vi "Apply Disabled.vi"(8 "error in (no error)":errorcluster, 10 "Disabled":bool, 11 "BluelinesRedlines in":refnum<class "BluelinesRedlines.lvclass">) -> (0 "error out":errorcluster, 3 "BluelinesRedlines out":refnum<class "BluelinesRedlines.lvclass">)   [LabVIEW 2020, in "VolatusGUIElements.lvlib" / "BluelinesRedlines.lvclass"]
uses:
  BluelinesRedlines.lvclass
  BluelinesRedlines.lvclass/BluelinesRedlines.ctl
  VolatusGUI/GUI Element/GUI Element.lvclass
  C:/dev/lv20CE/relink/lv-volatus/VolatusGUI/GUI Element/GUI Element.lvclass
  C:/dev/lv20CE/relink/lv-volatus/VolatusGUIElements/BluelinesRedlines/BluelinesRedlines.lvclass
  C:/dev/lv20CE/relink/lv-volatus/VolatusGUI/OnValueChangeHandler/OnValueChangeHandler.lvclass
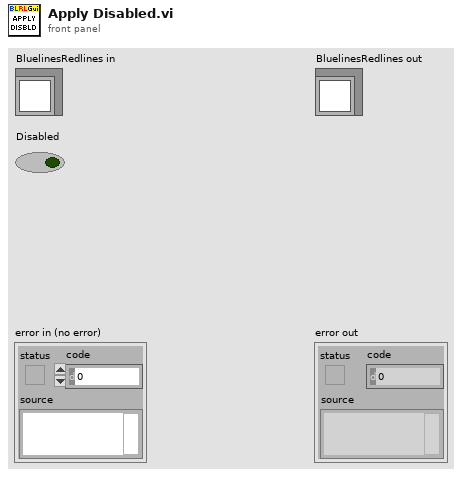
[diagram p1: front panel]
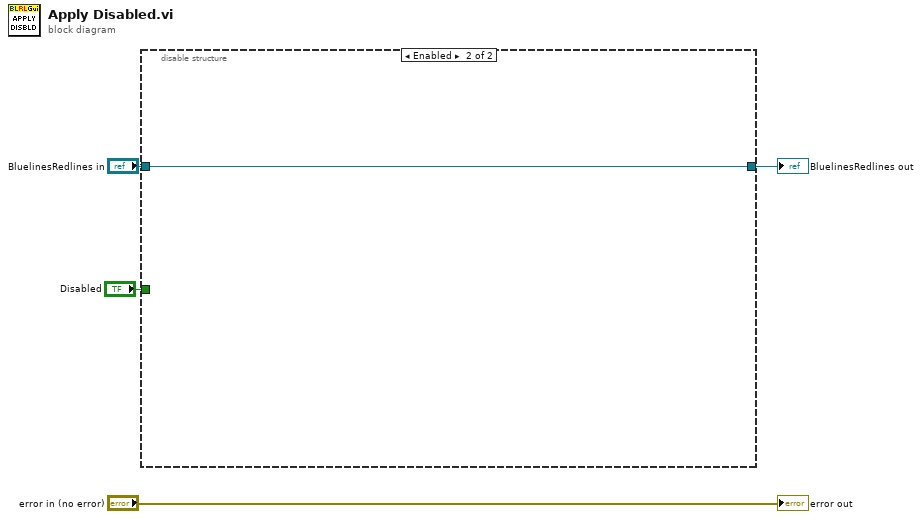
[diagram p0: block diagram]
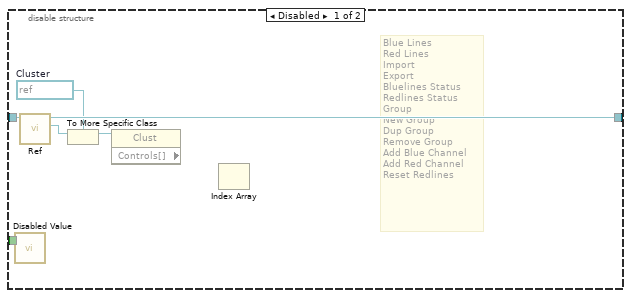
[diagram p2: hidden frame]
diagram:
  n1 = disable-structure shown="Enabled" {
    disable-tunnel: "BluelinesRedlines in" -> [w10 w11]
    disable-tunnel: "Disabled" -> [w9 _]
    disable-tunnel: [w8 w11] -> w1
    frame Disabled {
      w6 = refnum<vi> refnum  # Cluster
      # "Blue Lines\nRed Lines\nImport\nExport\nBluelines Status\nRedlines Status\nGroup\nNew Group\nDup Group\nRemove Group\nAdd Blue Channel\nAdd Red Channel\nReset Redlines"
      n2 = call "Disabled Value.vi"("Disabled"=w9) -> ()  [unwired: 6 in, 1 out]
      n3 = call "Ref.vi"("GUI Element in"=w10) -> ("Ref"=w7:refnum<vi>, "GUI Element out"=w8:refnum<class "BluelinesRedlines.lvclass">)  [unwired: 9 in]
      n4 = To More Specific Class(target class=w6, reference=w7) -> (specific class reference=w5:refnum<vi>)  [unwired: 1 in, 1 out]
      n5 = property class="Clust" props=["Controls[]"](reference=w5) -> ()  [unwired: 1 in, 3 out]
      n6 = Index Array() -> ()  [unwired: 2 in, 1 out]
    }
    frame Enabled {
    }
  }
  "BluelinesRedlines out" <- w1
  "error out" <- "error in (no error)"
